vi "Update Wash Entry Text.vi"(8 "error in (no error)":errorcluster, 10 "Wash Entry Text":string, 11 "Simulated Wash Display Console in":refnum<class "Simulated Wash Display Console.lvclass">) -> (0 "error out":errorcluster, 3 "Simulated Wash Display Console out":refnum<class "Simulated Wash Display Console.lvclass">)   [LabVIEW 2012, in "Simulated Wash Display Console.lvlib" / "Simulated Wash Display Console.lvclass"]
uses:
  Simulated Wash Display Console.lvclass
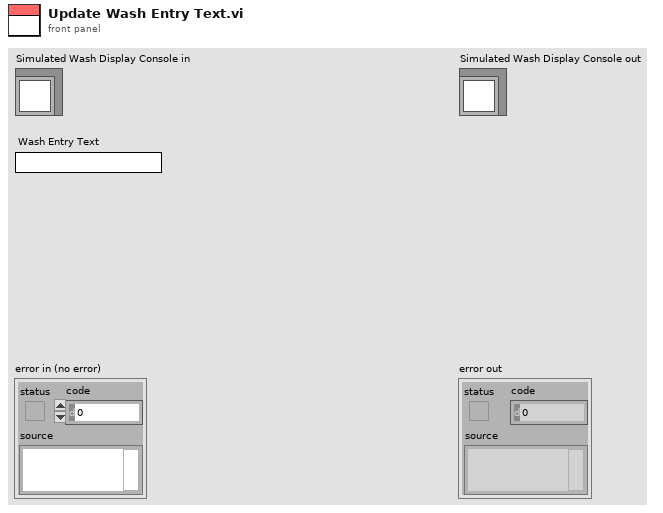
[diagram p1: front panel]
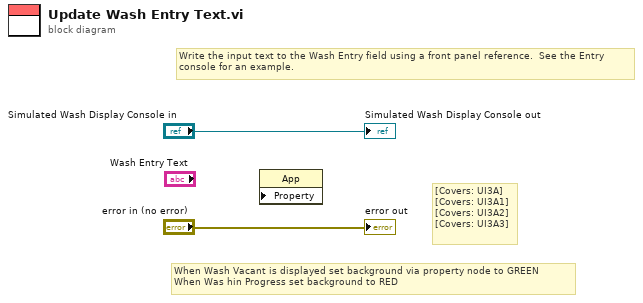
[diagram p0: block diagram]
diagram:
  # "When Wash Vacant is displayed set background via property node to GREEN\nWhen Was hin Progress set background to RED"
  # "[Covers: UI3A]\n[Covers: UI3A1]\n[Covers: UI3A2]\n[Covers: UI3A3]"
  # "Write the input text to the Wash Entry field using a front panel reference.  See the Entry\nconsole for an example."
  n1 = property class="App" props=[]() -> ()  [unwired: 3 in, 2 out]
  "error out" <- "error in (no error)"
  "Simulated Wash Display Console out" <- "Simulated Wash Display Console in"
